vi "IZGetPosition.vi"(0 "PRIORLib.IStageIn":refnum<k7>, 1 "error in (no error)":errorcluster) -> (2 "PRIORLib.IStageOut":refnum<k7>, 3 "error out":errorcluster, 4 "ZPos":dbl)   [LabVIEW 2011]
panel:
  # "This SubVi gets the Z axis position\nand returns immediately."
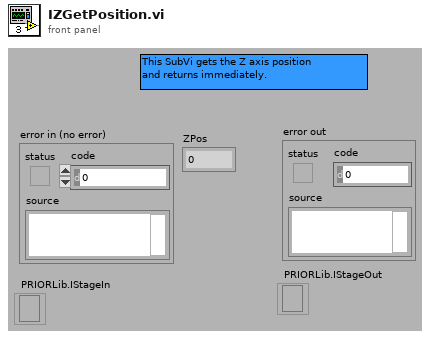
[diagram p1: front panel]
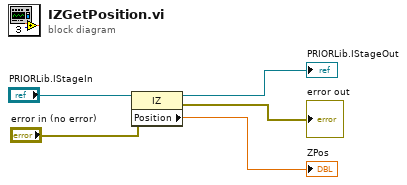
[diagram p0: block diagram]
diagram:
  n1 = property class="IZ"(reference="PRIORLib.IStageIn", error in="error in (no error)") -> (reference out=→"PRIORLib.IStageOut":refnum<k7>, error out=→"error out":errorcluster, "Position"=→"ZPos":dbl)
